vi "JSON Parse Command.vi"(8 "error in (no error)":errorcluster, 11 "JSON command":string) -> (0 "error out":errorcluster, 2 "key found?":bool, 3 "returned command":string)   [LabVIEW 2020, in "horiba.lvlib" / "Communicator.lvclass"]
doc: "Parses the original command."
uses:
  Communicator.lvclass
  49157962-a733-4a1d-a28f-690e3d97aae6.vi
  <vilib>/JDP Science/JSONtext/Find Item.vi
  <vilib>/JDP Science/JSONtext/Next JSON Value.vi
  <vilib>/JDP Science/JSONtext/String Subset.vi
  <vilib>/JDP Science/JSONtext/Parsing/Advance past next JSON Value (inlined COPY).vi
  <vilib>/JDP Science/JSONtext/Parsing/Advance past whitespace.vi
  <vilib>/JDP Science/JSONtext/Parsing/Advance past String.vi
  <vilib>/JDP Science/JSONtext/Parsing/Advance past Number.vi
  <vilib>/JDP Science/JSONtext/Parsing/Advance past Line Ending.vi
  <vilib>/JDP Science/JSONtext/Parsing/Parse Full Path or Item Name.vi
  <vilib>/JDP Science/JSONtext/Parsing/Advance past Array.vi
  <vilib>/JDP Science/JSONtext/Parsing/Advance past Object.vi
  <vilib>/JDP Science/JSONtext/support/Error Cluster From Code.vi
  <vilib>/JDP Science/JSONtext/Offset/Find Item Locations by Path.vi
  <vilib>/JDP Science/JSONtext/JSON text to Variant.vi
  <vilib>/JDP Science/JSONtext/LVClass Serializer/JSONtext LVClass Serializer.lvclass
panel:
  # "Connector Pane"
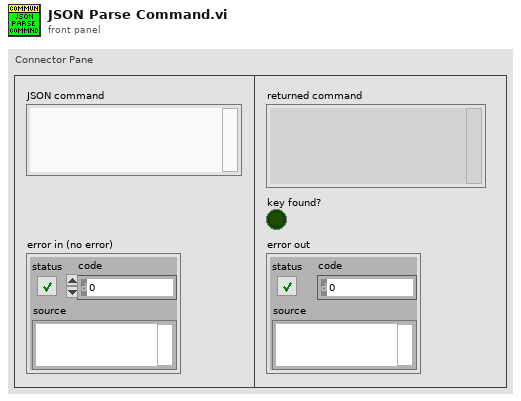
[diagram p1: front panel]
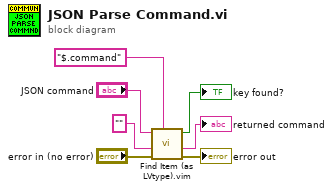
[diagram p0: block diagram]
diagram:
  n1 = call "Find Item (as LVtype).vim"("$Path or Item Name"="$.command", "error in (no error)"="error in (no error)", "Data Type and Default Value"="", "JSON"="JSON command") -> ("error out"=→"error out":errorcluster, "Data"=→"returned command":string, "Found"=→"key found?":bool)  [unwired: 4 in, 1 out]
